vi "IsEXE.vi"() -> (2 "path to vi or exe install\\data\\ dir":path, 5 "is exe?":bool)   [LabVIEW 2009]
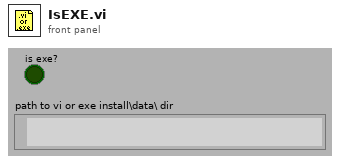
[diagram p1: front panel]
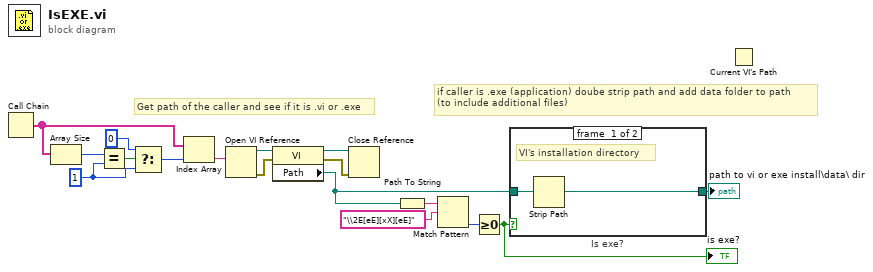
[diagram p0: block diagram]
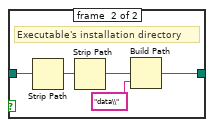
[diagram p2: hidden frame]
diagram:
  w9 = 1 ("index")
  # "if caller is .exe (application) doube strip path and add data folder to path\n(to include additional files)"
  # "Get path of the caller and see if it is .vi or .exe"
  n1 = Call Chain() -> (call chain=w13:string[])
  n2 = Array Size(array=w13) -> (size(s)=w10:i32)
  n3 = Equal?(x=w10, y=w9) -> (x = y?=w12:bool)
  n4 = Select(t=0, s=w12, f=w9) -> (s? t:f=w11:i32)
  n5 = Index Array(array=w13, index=w11) -> (element=w5:string)
  n6 = Open VI Reference(vi path=w5) -> (vi reference=w6:refnum<vi>, error out=w7:errorcluster)  [unwired: 1 in, 4 out]
  n7 = property class="VI"(reference=w6, error in=w7) -> (reference out=w2:refnum<vi>, error out=w3:errorcluster, "Path"=w4:path)
  n8 = Close Reference(reference=w2, error in (no error)=w3) -> ()  [unwired: 1 out]
  n9 = Path To String(path=w4) -> (string=w15:string)
  n10 = Match Pattern(string=w15, regular expression="\\2E[eE][xX][eE]") -> (offset past match=w16:i32)  [unwired: 4 out]
  n11 = Greater Or Equal To 0?(x=w16) -> (x >= 0?=w1:bool)
  "is exe?" <- w1
  n12 = case "Is exe?" shown="True" w1 {
    tunnel: w4 -> [w19 w24]
    tunnel: [w18 w21] -> w17
    frame #0 {
      # "VI's installation directory"
      n13 = Strip Path(path=w19) -> (stripped path=w18:path)  [unwired: 1 out]
    }
    frame #1 {
      # "Executable's installation directory"
      n14 = Strip Path(path=w24) -> (stripped path=w23:path)  [unwired: 1 out]
      n15 = Strip Path(path=w23) -> (stripped path=w22:path)  [unwired: 1 out]
      n16 = Build Path(base path=w22, name or relative path="data\\") -> (appended path=w21:path)
    }
  }
  "path to vi or exe install\\data\\ dir" <- w17
  n17 = Current VI's Path() -> ()  [unwired: 1 out]
